vi "LV_GetSysMetrics.vi"() -> (0 "UserMetrics":cluster{"UserWidth":i32, "UserHeight":i32}, 1 "SysMetrics":cluster{"FullWidth":i32, "FullHeight":i32}, 2 "Rect":T1, 3 "SM_CYSIZE":i32)   [LabVIEW 2015]
uses:
  C:/Windows/System32/user32.dll
panel:
  out "SM_CYFULLSCREEN":i32
  out "SM_CXFULLSCREEN":i32
  out "Height":i32
  out "Width":i32
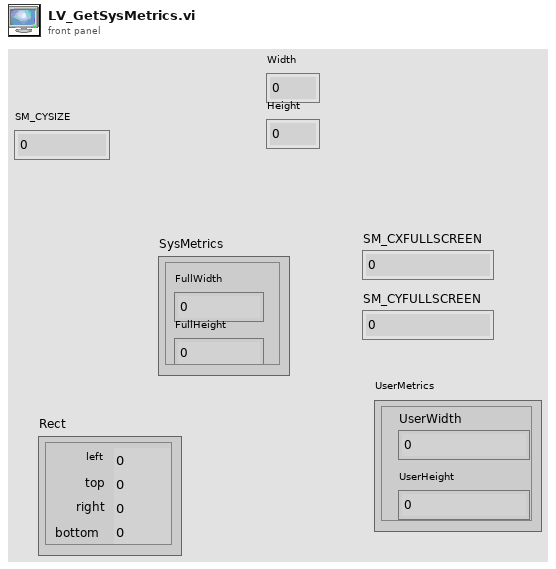
[diagram p1: front panel]
types:
  T1 = cluster{"left":i32, "top":i32, "right":i32, "bottom":i32}
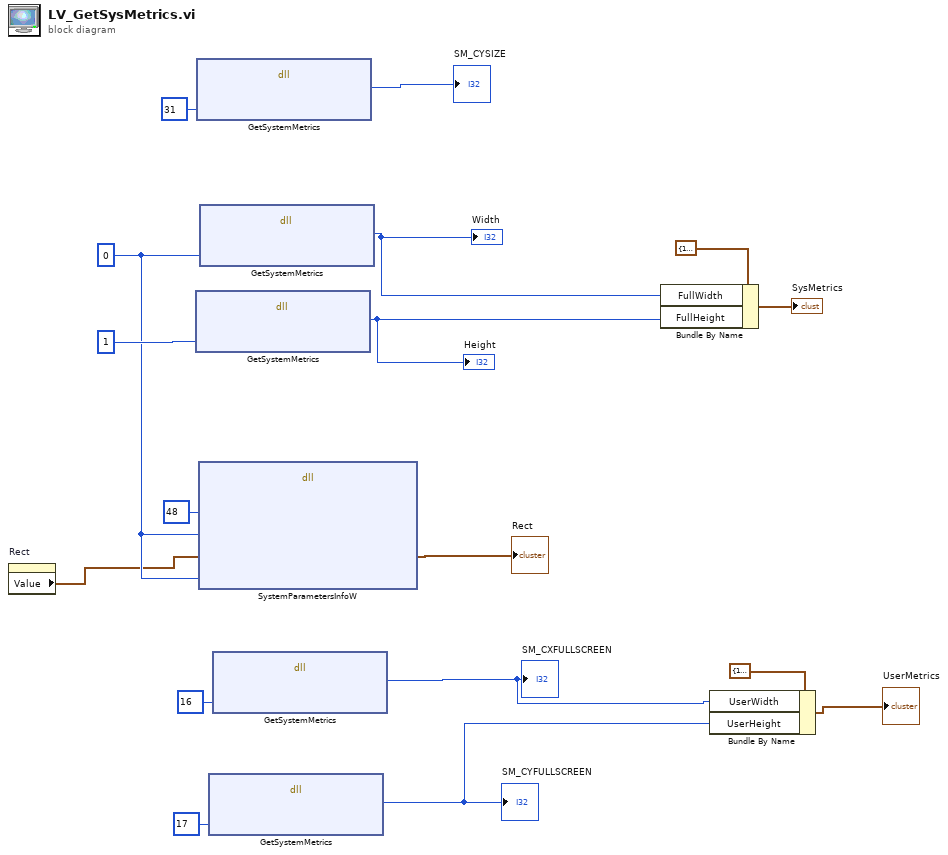
[diagram p0: block diagram]
diagram:
  w14 = 0 ("参数1")
  n1 = property on="Rect" class="Clust (严格)"() -> ("Value"=w10:T1)  [unwired: 2 in, 2 out]
  n2 = dll-call lib="C:/Windows/System32/user32.dll" fn="GetSystemMetrics"("ParaIndex"=1 ("参数1")) -> ("ScreenHeight"=w16:i32)  [unwired: 4 in, 2 out]
  "Height" <- w16
  n3 = dll-call lib="C:/Windows/System32/user32.dll" fn="GetSystemMetrics"("ParaIndex"=31) -> ("SM_CYSIZE"=→"SM_CYSIZE":i32)  [unwired: 4 in, 2 out]
  n4 = dll-call lib="C:/Windows/System32/user32.dll" fn="SystemParametersInfoW"("SPI_GETWORKAREA"=48, "null"=w14, "RT"=w10, "null"=w14) -> ("RT"=→"Rect":T1)  [unwired: 7 in, 2 out]
  n5 = dll-call lib="C:/Windows/System32/user32.dll" fn="GetSystemMetrics"("ParaIndex"=w14) -> ("ScreenWidth"=w17:i32)  [unwired: 4 in, 2 out]
  "Width" <- w17
  n6 = dll-call lib="C:/Windows/System32/user32.dll" fn="GetSystemMetrics"("ParaIndex"=17) -> ("SM_CYFULLSCREEN"=w4:i32)  [unwired: 4 in, 2 out]
  "SM_CYFULLSCREEN" <- w4
  n7 = dll-call lib="C:/Windows/System32/user32.dll" fn="GetSystemMetrics"("ParaIndex"=16) -> ("SM_CXFULLSCREEN"=w5:i32)  [unwired: 4 in, 2 out]
  "SM_CXFULLSCREEN" <- w5
  n8 = Bundle By Name(cluster=cluster{"FullWidth":i32, "FullHeight":i32} {"FullWidth"=1920, "FullHeight"=1080} ("SysMetrics"), "FullWidth"=w17, "FullHeight"=w16) -> (→"SysMetrics":cluster{"FullWidth":i32, "FullHeight":i32})
  n9 = Bundle By Name(cluster=cluster{"UserWidth":i32, "UserHeight":i32} {"UserWidth"=1827, "UserHeight"=1052} ("UserMetrics"), "UserWidth"=w5, "UserHeight"=w4) -> (→"UserMetrics":cluster{"UserWidth":i32, "UserHeight":i32})
